vi "Colour Items of a JSON string control.vi"(10 "String Control":refnum<vi>, 11 "JSON":string) -> ()   [LabVIEW 2015, in "JSONtext.lvlib"]
uses:
  JSONtext.lvlib
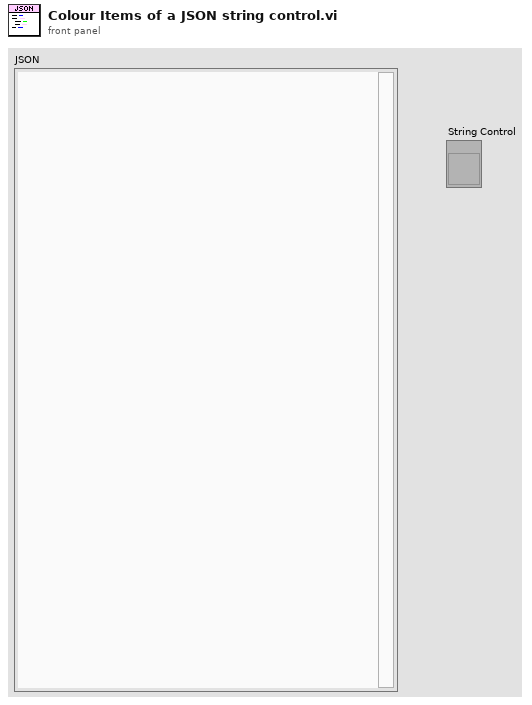
[diagram p1: front panel]
types:
  T1 = typedef "JSONtext.lvlib/JSON Value Type.ctl" = enum16{"Not a JSON Value", "JSON Object", "JSON Array", "String", "Number", "true", "false", "null"}
  T2 = cluster{"Value start out":i32, "Offset past match":i32, "JSON Value Type":T1}[]
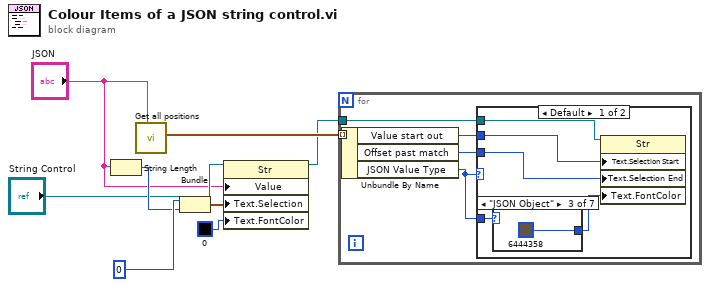
[diagram p0: block diagram]
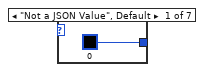
[diagram p2: hidden frame]
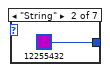
[diagram p3: hidden frame]
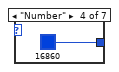
[diagram p4: hidden frame]
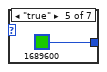
[diagram p5: hidden frame]
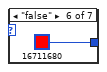
[diagram p6: hidden frame]
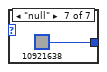
[diagram p7: hidden frame]
diagram:
  n1 = String Length(string="JSON") -> (length=w6:i32)
  n2 = call "Get all positions.vi"("JSON"="JSON") -> ("Array"=w8:T2)  [unwired: 8 in, 2 out]
  n3 = Bundle("Selection Start"=u32 0, w6) -> (w5:cluster{"Selection Start":u32, i32})  [unwired: 1 in]
  n4 = property on="Property Node" class="Str"(reference="String Control", "Value"="JSON", "Text.Selection"=w5, "Text.FontColor"=u32 0) -> (reference out=w3:refnum<vi>)  [unwired: 1 in, 1 out]
  n5 = for {
    tunnel: w8 -> [w13] mode=indexing
    tunnel: w3 -> [w9]
    n6 = Unbundle By Name(w13) -> ("Value start out"=w12:i32, "Offset past match"=w11:i32, "JSON Value Type"=w10:T1)
    n7 = case shown="Default" w10 {
      tunnel: w10 -> [w18 _]
      tunnel: w12 -> [w16 _]
      tunnel: w11 -> [w15 _]
      tunnel: w9 -> [w14 _]
      frame Default {
        n8 = case shown="\"JSON Object\"" w18 {
          tunnel: [u32 0 u32 12255432 u32 6444358 u32 16860 u32 1689600 u32 16711680 u32 10921638] -> w17
          frame "Not a JSON Value", Default {
          }
          frame "String" {
          }
          frame "JSON Object" {
          }
          frame "Number" {
          }
          frame "true" {
          }
          frame "false" {
          }
          frame "null" {
          }
        }
        n9 = property on="Property Node" class="Str"(reference=w14, "Text.Selection Start"=w16, "Text.Selection End"=w15, "Text.FontColor"=w17) -> ()  [unwired: 1 in, 2 out]
      }
      frame "JSON Object" {
      }
    }
  }
